vi "flow-builder-irrigation-dose.vi"(10 "Digital Timeout":u16, 11 "OUTPUT(+AUX)":string[](array[string])) -> (3 "Flow":T1[](array[typedef]))   [LabVIEW 2024]
uses:
  controls/UiStepBuilder.ctl
  controls/type.step-builder.ctl
panel:
  in  "Unit Index":i32
  in  "Proc Name (empty: bypass logging)":string="UNIT%d"
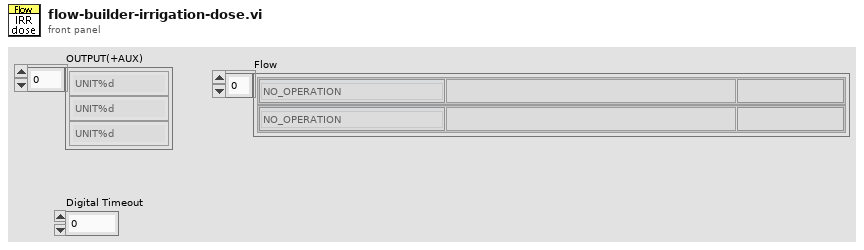
[diagram p1: front panel]
types:
  T1 = typedef "UiStepBuilder.ctl" = cluster{"Step Function":T2, "ParamString":string, "Step Label":string}
  T2 = typedef "type.step-builder.ctl" = enum16{"NO_OPERATION", "DELAY-JUMP", "DELAY", "JUMP", "COMPLETE", "SCHEDULER", "IRR-CHECK", "UNIT-CHECK", "UNIT-SAMPLE", "UNIT-DOSE", "LOG-REPORT", "LOG-MESSAGE", "IO-READ", "IO-READ-MANY", "IO-WRITE", "IO-COMPARE-OUT", "IO-COMPARE-IN", "PROC-START", "PROC-STOP", "PROC-LOAD", "PROC-IS-COMPLETED", "RECORD-MOVE", "GET-RH", "GET-UV", "GET-WD", "GET-WS", "OCS-CHECK", "OCS-RECORD"}
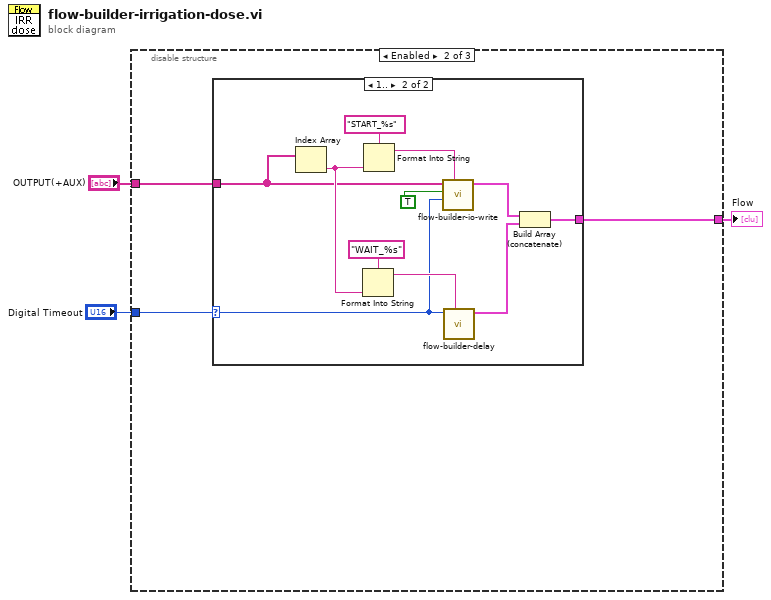
[diagram p0: block diagram]
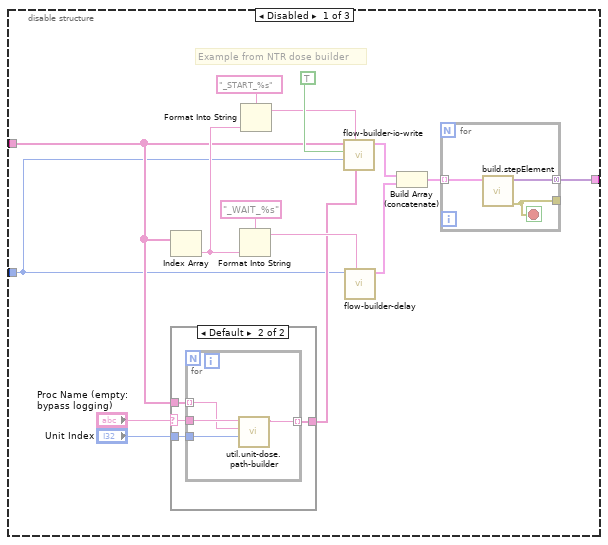
[diagram p2: hidden frame]
diagram:
  n1 = disable-structure shown="Enabled" {
    disable-tunnel: [w18 w31 _] -> w3
    disable-tunnel: "OUTPUT(+AUX)" -> [w8 w32 _]
    disable-tunnel: "Digital Timeout" -> [w4 w30 _]
    frame Disabled {
      # "Example from NTR dose builder"
      n2 = Index Array(array=w8) -> (element=w10:string)  [unwired: 1 in]
      n3 = case shown="Default" "Proc Name (empty: bypass logging)" {
        selector: "Proc Name (empty: bypass logging)" -> [_ w21]
        tunnel: w8 -> [_ w22]
        tunnel: "Unit Index" -> [_ w20]
        tunnel: [_ w19] -> w5
        frame "False" {
        }
        frame Default {
          n4 = for {
            tunnel: w22 -> [w25] mode=indexing
            tunnel: w21 -> [w26]
            tunnel: w20 -> [w24]
            tunnel: [w23] -> w19 mode=indexing
            n5 = call "util.unit-dose.path-builder.vi"("Unit Index"=w24, "Input"=w25, "Proc Name"=w26) -> ("\\NUTRITION\\ORP\\ORP_U1_2024-08-16.*"=w23:string)  [unwired: 8 in]
          }
        }
      }
      n6 = Format Into String(format string="_WAIT_%s", w10) -> (resulting string=w12:string)  [unwired: 2 in, 1 out]
      n7 = Format Into String(format string="_START_%s", w10) -> (resulting string=w9:string)  [unwired: 2 in, 1 out]
      n8 = call "flow-builder-io-write.vi"("filenames.*"=w5, "Step Name"=w9, "Digital Timeout"=w4, "Value in"=TRUE, "Dout+AUX"=w8) -> ("Flow out"=w16:T1[])  [unwired: 6 in]
      n9 = call "flow-builder-delay.vi"("Step Label"=w12, "Delay [s]"=w4) -> ("Step Element"=w15:T1)  [unwired: 9 in]
      n10 = Build Array (concatenate)(w16, w15) -> (w14:T1[])
      n11 = for {
        tunnel: w14 -> [w29] mode=indexing
        tunnel: [w28] -> w18 mode=concatenating
        tunnel: [w27] -> _
        stop <- w27 stop-if-true
        n12 = call "build.stepElement.vi"("Step in"=w29) -> ("error out"=w27:errorcluster, "steps out"=w28:variant[])  [unwired: 9 in]
      }
    }
    frame Enabled {
      n13 = case shown="1.." w30 {
        selector: w30 -> [_ w33]
        tunnel: w32 -> [_ w35]
        tunnel: [_ w34] -> w31
        frame 0, Default {
        }
        frame 1.. {
          n14 = Index Array(array=w35) -> (element=w37:string)  [unwired: 1 in]
          n15 = Format Into String(format string="WAIT_%s", w37) -> (resulting string=w39:string)  [unwired: 2 in, 1 out]
          n16 = Format Into String(format string="START_%s", w37) -> (resulting string=w36:string)  [unwired: 2 in, 1 out]
          n17 = call "flow-builder-io-write.vi"("Step Name"=w36, "Digital Timeout"=w33, "Value in"=TRUE, "Dout+AUX"=w35) -> ("Flow out"=w42:T1[])  [unwired: 7 in]
          n18 = call "flow-builder-delay.vi"("Step Label"=w39, "Delay [s]"=w33) -> ("Step Element"=w41:T1)  [unwired: 9 in]
          n19 = Build Array (concatenate)(w42, w41) -> (w34:T1[])
        }
      }
    }
    frame Disabled {
    }
  }
  "Flow" <- w3
